vi "Sub Pic Build Bitmap.vi"(9 "Height":i16, 10 "Width":i16, 11 "RGB Array":cluster{"R":u8, "G":u8, "B":u8}[](array[cluster])) -> (3 "24-bit pixmap (RGB)":u32[][](array[numeric]) format="%x")   [LabVIEW 2018, in "Picture Process.lvclass"]
uses:
  Picture Process.lvclass
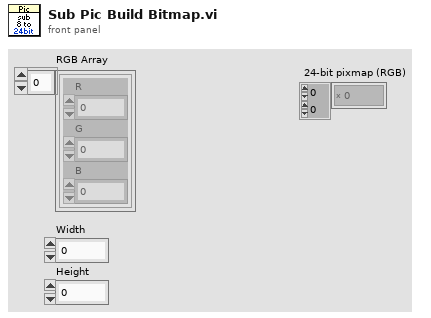
[diagram p1: front panel]
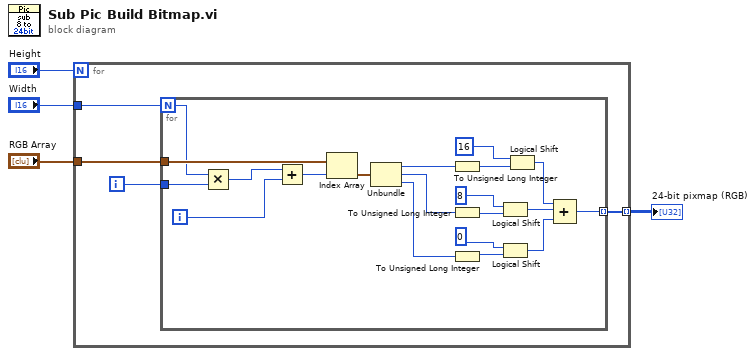
[diagram p0: block diagram]
diagram:
  n1 = for {
    N: "Height" -> [_]
    tunnel: "Width" -> [w7]
    tunnel: [w8] -> w1 mode=indexing
    tunnel: "RGB Array" -> [w6]
    i -> [w5]
    n2 = for {
      N: w7 -> [w10]
      tunnel: [w22] -> w8 mode=indexing
      tunnel: w6 -> [w18]
      tunnel: w5 -> [w11]
      i -> [w12]
      n3 = Multiply(x=w10, y=w11) -> (x*y=w9:i32)
      n4 = Add(x=w9, y=w12) -> (x+y=w13:i32)
      n5 = Index Array(array=w18, index=w13) -> (element=w17:cluster{"R":u8, "G":u8, "B":u8})
      n6 = Unbundle(w17) -> ("R"=w16:u8, "G"=w15:u8, "B"=w14:u8)
      n7 = To Unsigned Long Integer(number=w16) -> (unsigned 32bit integer=w20:u32)
      n8 = To Unsigned Long Integer(number=w15) -> (unsigned 32bit integer=w26:u32)
      n9 = To Unsigned Long Integer(number=w14) -> (unsigned 32bit integer=w25:u32)
      n10 = Logical Shift(y=i8 8, x=w26) -> (x << y=w24:u32)
      n11 = Logical Shift(y=i8 0, x=w25) -> (x << y=w23:u32)
      n12 = Logical Shift(y=i8 16, x=w20) -> (x << y=w19:u32)
      n13 = Compound Arithmetic op=ADD(w19, w24, w23) -> (w22:u32)
    }
  }
  "24-bit pixmap (RGB)" <- w1
